vi "Disconnect OPC UA.vi"(8 "error in (no error)":errorcluster, 10 "OPC UA refnum":T1, 11 "OPC UA In":refnum<class "OPC UA.lvclass">) -> (0 "error out":errorcluster, 3 "OPC UA out":refnum<class "OPC UA.lvclass">)   [LabVIEW 2019, in "OPC UA.lvlib" / "OPC UA.lvclass"]
uses:
  OPC UA.lvclass
  OPC UA.lvclass/OPC UA.ctl
  <vilib>/OPCUA/NI OPC UA Client.lvlib
  <vilib>/OPCUA/controls/OPC UA Client Refnum.ctl
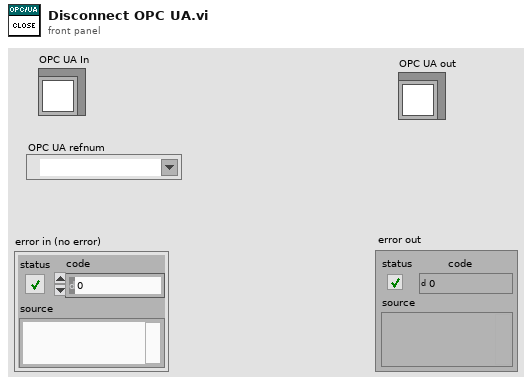
[diagram p1: front panel]
types:
  T1 = typedef "OPC UA Client Refnum.ctl" = refnum<k21>
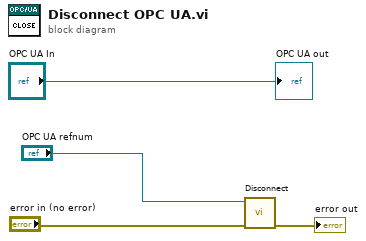
[diagram p0: block diagram]
diagram:
  n1 = call <vilib>:"Disconnect.vi"("error in (no error)"="error in (no error)", "OPC UA client refnum in"="OPC UA refnum") -> ("error out"=→"error out":errorcluster)  [unwired: 9 in]
  "OPC UA out" <- "OPC UA In"
